vi "ADconverter.vi"(1 "resolution (16 bit)":i32=16, 2 "Analog signal":waveform(dbl)) -> (0 "Digital signal":dbl[](array[numeric]))   [LabVIEW 2013]
uses:
  <vilib>/Waveform/DWDTOps.llb/DWDT Analog to Digital.vi
  <vilib>/Waveform/DTblOps.llb/DTbl Digital to Boolean Array.vi
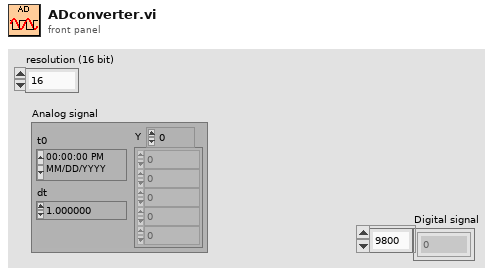
[diagram p1: front panel]
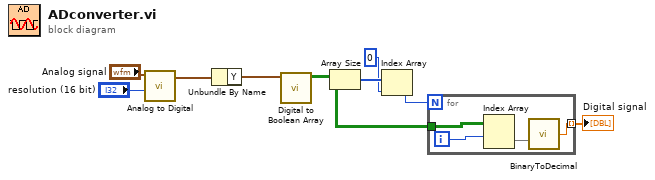
[diagram p0: block diagram]
diagram:
  n1 = call-poly <vilib>:"Analog to Digital.vi"("resolution (16 bit)"="resolution (16 bit)", "analog waveform"="Analog signal") -> ("digital waveform"=w3:digitalwaveform)  [unwired: 6 in, 3 out]
  n2 = Unbundle By Name(w3) -> ("Y"=w2:digitaldata)
  n3 = call-poly <vilib>:"Digital to Boolean Array.vi"("digital data"=w2) -> ("boolean array"=w1:bool[][])  [unwired: 9 in, 1 out]
  n4 = Array Size(array=w1) -> (size(s)=w8:i32[])
  n5 = Index Array(array=w8, index=0) -> (element=w5:i32)
  n6 = for {
    N: w5 -> [_]
    tunnel: w1 -> [w13]
    tunnel: [w10] -> w4 mode=indexing
    i -> [w12]
    n7 = Index Array(array=w13, index (row)=w12) -> (element=w11:bool[])  [unwired: 1 in]
    n8 = call "BinaryToDecimal.vi"("Binary"=w11) -> ("Decimal"=w10:dbl)  [unwired: 2 in]
  }
  "Digital signal" <- w4
